vi "Command.vi"(5 "success response (\\06)":string="\u0006", 7 "additional timeout, ms (0)":u32, 8 "error in (no error)":errorcluster, 9 "data":i32=-1, 10 "command":string, 11 "SOL MS in":refnum<class "PL SOL Instruments MS.lvclass">) -> (0 "error out":errorcluster, 3 "SOL MS out":refnum<class "PL SOL Instruments MS.lvclass">)   [LabVIEW 2015, in "PL SOL Instruments MS.lvclass"]
doc: "Sends <b>command</b> to device and returns <b>response data</b>."
uses:
  PL SOL Instruments MS.lvclass
  PL SOL Instruments MS.lvclass/PL SOL Instruments MS.ctl
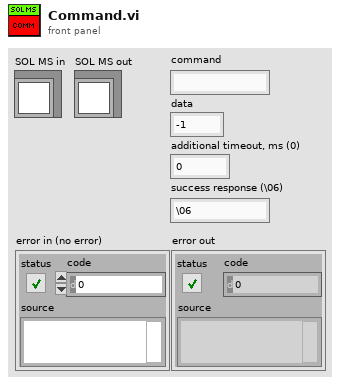
[diagram p1: front panel]
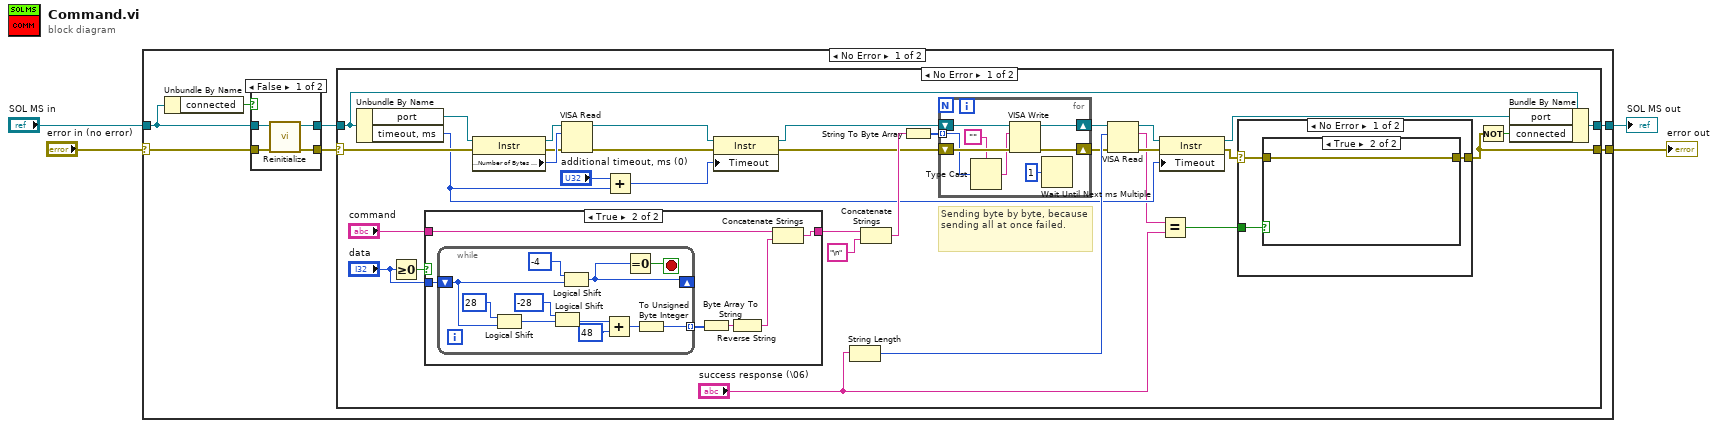
[diagram p0: block diagram]
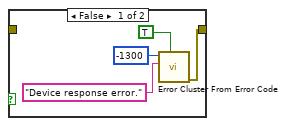
[diagram p2: hidden frame]
diagram:
  n1 = case shown="No Error" "error in (no error)" {
    selector: "error in (no error)" -> [w9 w89]
    tunnel: "SOL MS in" -> [w10 w88]
    tunnel: [w6 w89] -> w1
    tunnel: [w5 w88] -> w2
    frame No Error {
      n2 = Unbundle By Name(w10) -> ("connected"=w11:bool)
      n3 = case shown="False" w11 {
        tunnel: w10 -> [w85 w87]
        tunnel: w9 -> [w84 w86]
        tunnel: [w83 w87] -> w7
        tunnel: [w82 w86] -> w8
        frame False {
          n4 = call "Reinitialize.vi"("error in (no error)"=w84, "SOL MS in"=w85) -> ("error out"=w82:errorcluster, "SOL MS out"=w83:refnum<class "PL SOL Instruments MS.lvclass">)  [unwired: 8 in]
        }
        frame True {
        }
      }
      n5 = case shown="No Error" w8 {
        selector: w8 -> [w38 w81]
        tunnel: w7 -> [w44 w80]
        tunnel: [w13 w81] -> w6
        tunnel: [w42 w80] -> w5
        frame No Error {
          # "Sending byte by byte, because sending all at once failed."
          n6 = Unbundle By Name(w44) -> ("port"=w39:refnum<visa-resource-name>, "timeout, ms"=w18:u32)
          n7 = Greater Or Equal To 0?(x="data") -> (x >= 0?=w32:bool)
          n8 = case shown="True" w32 {
            tunnel: "command" -> [w62 w64]
            tunnel: "data" -> [_ w66]
            tunnel: [w62 w65] -> w35
            frame False {
            }
            frame True {
              n9 = while {
                shift-right: [w77] -> _
                shift-left: w66 -> [w76]
                tunnel: [w69] -> w68 mode=indexing
                stop <- w78 stop-if-true
                n10 = Logical Shift(y=28, x=w76) -> (x << y=w75:i32)
                n11 = Logical Shift(y=-28, x=w75) -> (x << y=w72:i32)
                n12 = Logical Shift(y=i16 -4, x=w76) -> (x << y=w77:i32)
                n13 = Add(x=w72, y=u32 48) -> (x+y=w70:u32)
                n14 = Equal To 0?(x=w77) -> (x = 0?=w78:bool)
                n15 = To Unsigned Byte Integer(number=w70) -> (unsigned 8bit integer=w69:u8)
              }
              n16 = Byte Array To String(unsigned byte array=w68) -> (string=w67:string)
              n17 = Reverse String(1:w67) -> (0:w63:string)
              n18 = Concatenate Strings(w64, w63) -> (w65:string)
            }
          }
          n19 = property class="Instr"(reference=w39, error in=w38) -> (reference out=w40:refnum<visa-resource-name>, error out=w37:errorcluster, "Serial Settings:Number of Bytes at Serial Port"=w41:u32)
          n20 = VISA Read(VISA resource name=w40, byte count=w41, error in (no error)=w37) -> (VISA resource name out=w27:refnum<visa-resource-name>, error out=w29:errorcluster)  [unwired: 2 out]
          n21 = Add(x="additional timeout, ms (0)", y=w18) -> (x+y=w28:u32)
          n22 = property class="Instr"(reference=w27, error in=w29, "Timeout"=w28) -> (reference out=w26:refnum<visa-resource-name>, error out=w25:errorcluster)
          n23 = String Length(string="success response (\\06)") -> (length=w24:i32)
          n24 = Concatenate Strings(w35, "\n" ("string")) -> (w31:string)
          n25 = String To Byte Array(string=w31) -> (unsigned byte array=w12:u8[])
          n26 = for {
            tunnel: w12 -> [w48] mode=indexing
            shift-right: [w50] -> w23
            shift-left: w26 -> [w52]
            shift-right: [w49] -> w22
            shift-left: w25 -> [w51]
            n27 = Type Cast(type="", x=w48) -> (*(type *) &x=w46:string)
            n28 = VISA Write(VISA resource name=w52, write buffer=w46, error in (no error)=w51) -> (VISA resource name out=w50:refnum<visa-resource-name>, error out=w49:errorcluster)  [unwired: 1 out]
            n29 = Wait Until Next ms Multiple(millisecond multiple=u32 1) -> ()  [unwired: 1 out]
          }
          n30 = VISA Read(VISA resource name=w23, byte count=w24, error in (no error)=w22) -> (VISA resource name out=w20:refnum<visa-resource-name>, read buffer=w16:string, error out=w21:errorcluster)  [unwired: 1 out]
          n31 = property class="Instr"(reference=w20, error in=w21, "Timeout"=w18) -> (reference out=w19:refnum<visa-resource-name>, error out=w17:errorcluster)
          n32 = Equal?(x=w16, y="success response (\\06)") -> (x = y?=w14:bool)
          n33 = case shown="No Error" w17 {
            selector: w17 -> [w54 w61]
            tunnel: [w55 w61] -> w13
            tunnel: w14 -> [w53 _]
            frame No Error {
              n34 = case shown="True" w53 {
                tunnel: [w56 w60] -> w55
                tunnel: w54 -> [_ w60]
                frame False {
                  n35 = call <vilib>:"Error Cluster From Error Code.vi"("show call chain? (False)"=TRUE, "error message (\"\")"="Device response error." ("error message (\"\")"), "error code (0)"=-1300) -> ("error out"=w56:errorcluster)  [unwired: 6 in]
                }
                frame True {
                }
              }
            }
            frame Error {
            }
          }
          n36 = Not(x=w13) -> (.not. x?=w43:bool)
          n37 = Bundle By Name(cluster=w44, "port"=w19, "connected"=w43) -> (w42:refnum<class "PL SOL Instruments MS.lvclass">)
        }
        frame Error {
        }
      }
    }
    frame Error {
    }
  }
  "SOL MS out" <- w2
  "error out" <- w1
